vi "Read Bit.vi"(8 "error in (no error)":errorcluster, 11 "Bit in":refnum<class "Bit.lvclass">) -> (0 "error out":errorcluster, 2 "Bit":bool, 3 "Bit out":refnum<class "Bit.lvclass">)   [LabVIEW 2016, in "Bit.lvclass"]
uses:
  Bit.lvclass
  Bit.lvclass/Bit.ctl
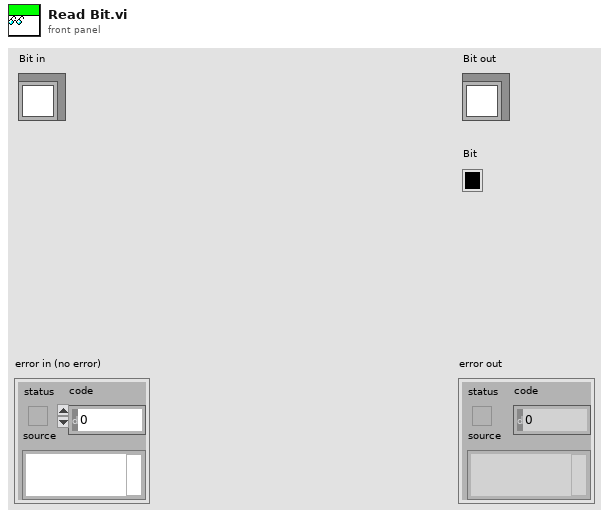
[diagram p1: front panel]
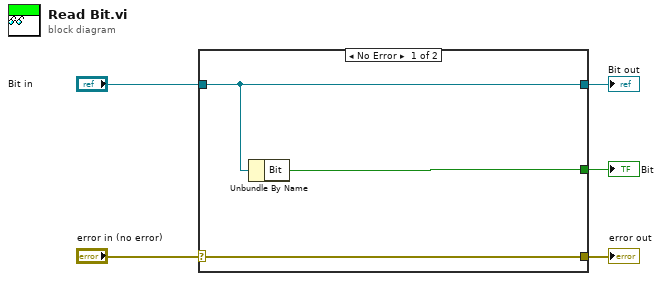
[diagram p0: block diagram]
diagram:
  n1 = case shown="No Error" "error in (no error)" {
    selector: "error in (no error)" -> [w8 w9]
    tunnel: [w8 w9] -> w4
    tunnel: [w7 w10] -> w2
    tunnel: "Bit in" -> [w7 w10]
    tunnel: [w6 _] -> w1
    frame No Error {
      n2 = Unbundle By Name(w7) -> ("Bit"=w6:bool)
    }
    frame Error {
    }
  }
  "error out" <- w4
  "Bit out" <- w2
  "Bit" <- w1
